vi "Configure Module.vi"(8 "error in (no error)":errorcluster, 10 "IOV ref in":refnum<k21>, 11 "9224 in":refnum<class "9224.lvclass">) -> (0 "error out":errorcluster, 2 "IOV ref out":refnum<k21>, 3 "9224 out":refnum<class "9224.lvclass">)   [LabVIEW 2019, in "Modules.lvlib" / "9224.lvclass"]
uses:
  9224.lvclass
  C:/Users/nitest/Desktop/Git 2019/niveristand-scan-engine-module-libraries/Source/RSI Module/RSI Module.lvclass
  9224.lvclass/9224.ctl
  <resource>/objmgr/cRIO.rc
  RSI Module/RSI Module.lvclass
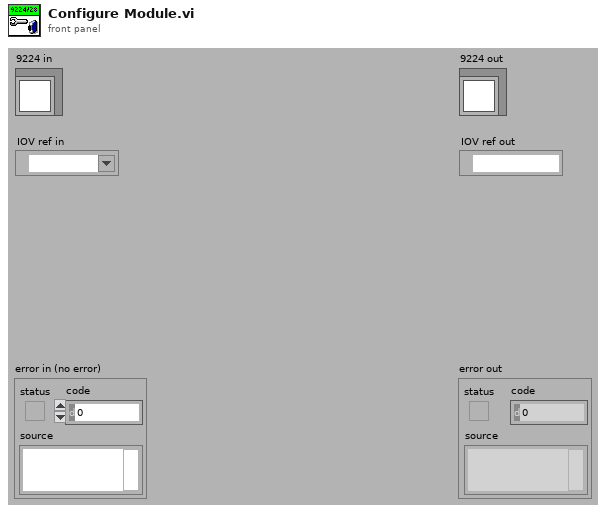
[diagram p1: front panel]
types:
  T1 = typedef "Modules.lvlib/9224.lvclass/Conversion Time.ctl" = u16
  T2 = typedef "Modules.lvlib/RSI Module.lvclass/Module Models.ctl" = enum16{"Empty", "NI 9201", "NI 9203", "NI 9205", "NI 9206", "NI 9207", "NI 9208", "NI 9209", "NI 9210", "NI 9211", "NI 9212", "NI 9213", "NI 9214", "NI 9215", "NI 9216", "NI 9217", "NI 9219", "NI 9220", "NI 9221", "NI 9222", "NI 9223", "NI 9224", "NI 9225", "NI 9226", "NI 9227", "NI 9228", "NI 9229", "NI 9233", "NI 9234", "NI 9235", "NI 9236", "NI 9237", "NI 9239", "NI 9242", "NI 9244", "NI 9253", "NI 9263", "NI 9264", "NI 9265", "NI 9266", "NI 9269", "NI 9344", "NI 9350", "NI 9375", "NI 9401", "NI 9402", "NI 9403", "NI 9411", "NI 9421", "NI 9422", "NI 9423", "NI 9425", "NI 9426", "NI 9435", "NI 9436", "NI 9437", "NI 9472", "NI 9474", "NI 9475", "NI 9476", "NI 9477", "NI 9478", "NI 9481", "NI 9482", "NI 9485"}
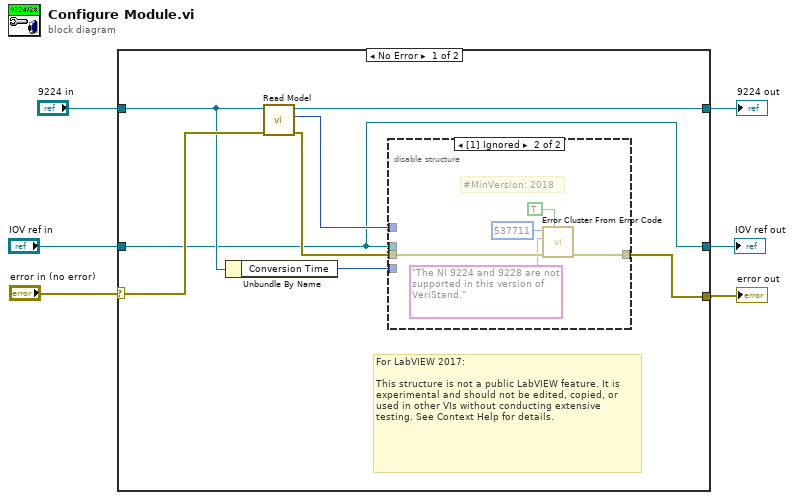
[diagram p0: block diagram]
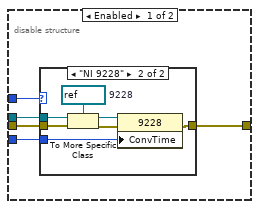
[diagram p2: hidden frame]
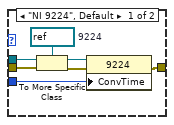
[diagram p3: hidden frame]
diagram:
  n1 = case shown="No Error" "error in (no error)" {
    selector: "error in (no error)" -> [w13 w41]
    tunnel: [w7 w41] -> w3
    tunnel: [w14 w40] -> w1
    tunnel: "9224 in" -> [w12 w40]
    tunnel: "IOV ref in" -> [w9 w39]
    tunnel: [w9 w39] -> w2
    frame No Error {
      # "For LabVIEW 2017:\n\nThis structure is not a public LabVIEW feature. It is experimental and should not be edited, copied, or used in other VIs without conducting extensive testing. See Context Help for details."
      n2 = Unbundle By Name(w12) -> ("Conversion Time"=w8:T1)
      n3 = call "Read Model.vi"("error in (no error)"=w13, "RSI Module in"=w12) -> ("error out"=w10:errorcluster, "Model"=w11:T2, "RSI Module out"=w14:refnum<class "9224.lvclass">)  [unwired: 7 in]
      n4 = disable-structure shown="[1] Ignored" {
        disable-tunnel: w11 -> [w19 _]
        disable-tunnel: w10 -> [w18 w37]
        disable-tunnel: w9 -> [w17 _]
        disable-tunnel: w8 -> [w16 _]
        disable-tunnel: [w15 w38] -> w7
        frame Enabled {
          n5 = case shown="\"NI 9228\"" w19 {
            tunnel: w18 -> [w26 w27]
            tunnel: [w22 w28] -> w15
            tunnel: w17 -> [w21 w29]
            tunnel: w16 -> [w20 w31]
            frame "NI 9224", Default {
              w25 = refnum<k21> refnum  # 9224
              n6 = To More Specific Class(target class=w25, reference=w21, error in=w26) -> (specific class reference=w24:refnum<k21>, error out=w23:errorcluster)
              n7 = property class="9224"(reference=w24, error in=w23, "ConvTime"=w20) -> (error out=w22:errorcluster)  [unwired: 1 out]
            }
            frame "NI 9228" {
              w30 = refnum<k21> refnum  # 9228
              n8 = To More Specific Class(target class=w30, reference=w29, error in=w27) -> (specific class reference=w33:refnum<k21>, error out=w32:errorcluster)
              n9 = property class="9228"(reference=w33, error in=w32, "ConvTime"=w31) -> (error out=w28:errorcluster)  [unwired: 1 out]
            }
          }
        }
        frame Disabled {
          # "#MinVersion: 2018"
          n10 = call <vilib>:"Error Cluster From Error Code.vi"("show call chain? (False)"=TRUE, "error in (no error)"=w37, "error message (\"\")"="The NI 9224 and 9228 are not supported in this version of VeriStand." ("error message (\"\")"), "error code (0)"=537711) -> ("error out"=w38:errorcluster)  [unwired: 5 in]
        }
      }
    }
    frame Error {
    }
  }
  "error out" <- w3
  "9224 out" <- w1
  "IOV ref out" <- w2
